vi "api_installation_test.vi"() -> ()   [LabVIEW 2017]
uses:
  C:/Users/Sameer/Documents/API/030620/AOL_API.dll
panel:
  out "API Exec time (ms)":u32
  out "input_array":dbl[][](array[numeric])
  out "return":i32
  out "output_matrix":dbl[][](array[numeric])
  in  "Element_value":dbl=2.5
  out "error out":errorcluster
  in  "error in (no error)":errorcluster
  in  "dim2":i32=7
  in  "dim1":i32=5
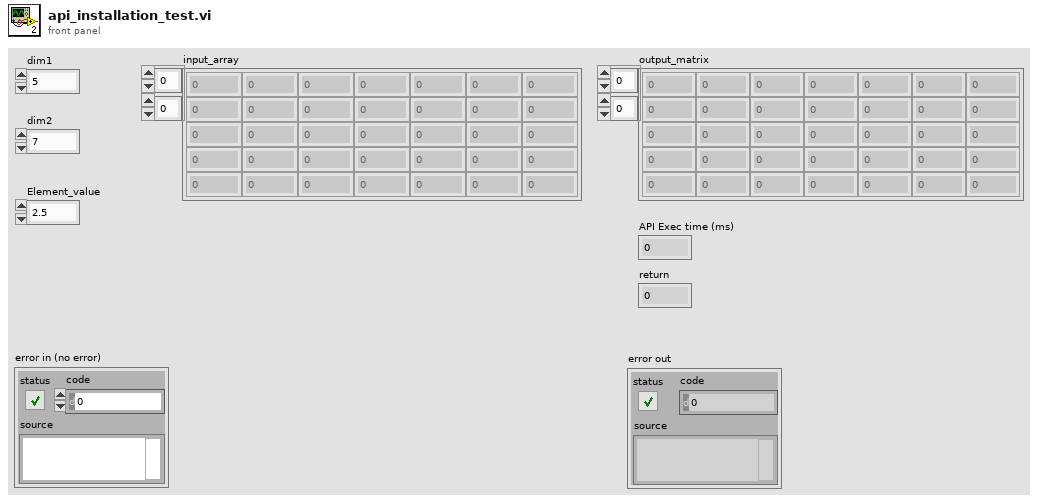
[diagram p1: front panel]
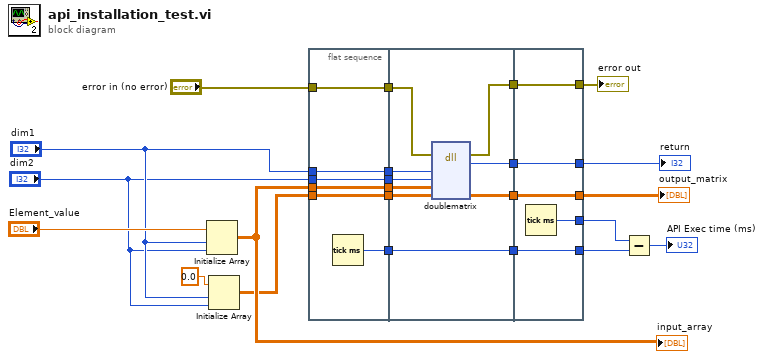
[diagram p0: block diagram]
diagram:
  n1 = Initialize Array("Element_value", "dim1", "dim2") -> (w22:dbl[][])
  "input_array" <- w22
  n2 = Initialize Array(0.0 ("element"), "dim1", "dim2") -> (w17:dbl[][])
  n3 = flat-sequence {
    tunnel: "error in (no error)" -> [w25]
    tunnel: w17 -> [w26]
    tunnel: "dim2" -> [w27]
    tunnel: "dim1" -> [w28]
    tunnel: w22 -> [w29]
    tunnel: [w29] -> w13
    tunnel: [w28] -> w12
    tunnel: [w27] -> w11
    tunnel: [w26] -> w10
    tunnel: [w25] -> w9
    tunnel: [w24] -> w4
    tunnel: w13 -> [w38]
    tunnel: w12 -> [w36]
    tunnel: w11 -> [w35]
    tunnel: w10 -> [w34]
    tunnel: w9 -> [w32]
    tunnel: [w37] -> w8
    tunnel: [w33] -> w7
    tunnel: [w31] -> w6
    tunnel: w4 -> [w30]
    tunnel: [w30] -> w3
    tunnel: [w41] -> w14
    tunnel: [w42] -> w16
    tunnel: [w43] -> w21
    tunnel: w8 -> [w43]
    tunnel: w7 -> [w42]
    tunnel: w6 -> [w41]
    tunnel: [w40] -> w5
    tunnel: w3 -> [w39]
    tunnel: [w39] -> w2
    frame #0 {
      n4 = Tick Count (ms)() -> (millisecond timer value=w24:u32)
    }
    frame #1 {
      n5 = dll-call lib="C:/Users/Sameer/Documents/API/030620/AOL_API.dll" fn="doublematrix"(error in=w32, "dim1"=w36, "dim2"=w35, "input_array"=w38, "output_array"=w34) -> (error out=w31:errorcluster, "return type"=w33:i32, "output_array"=w37:dbl[][])  [unwired: 5 in, 1 out]
    }
    frame #2 {
      n6 = Tick Count (ms)() -> (millisecond timer value=w40:u32)
    }
  }
  n7 = Subtract(x=w5, y=w2) -> (x-y=→"API Exec time (ms)":u32)
  "error out" <- w14
  "output_matrix" <- w21
  "return" <- w16
